vi "poly_asynch_wait_wait.vi"(4 "restart asynch wait? (F)":bool, 6 "check interval (50 ms)":u32=50, 8 "error in":errorcluster, 9 "timeout [ms]":i32, 10 "asynch wait ref in":T1) -> (0 "error out":errorcluster, 1 "timed out?":bool, 2 "asynch wait ref out":T1, 5 "remaining time":i32)   [LabVIEW 2015, in "_timing_tools_polys.lvlib"]
uses:
  _timing_tools_polys.lvlib
  asynch_wait_ref.ctl
  boolean_notifier.ctl
  poly_timing_tools_eco_plus.vi
  <vilib>/GPower/Timing/Library/Remaining/Remaining_ms.vi
  <vilib>/GPower/Timing/Library/Wait/Wait_ms.vi
  <vilib>/GPower/Error/Library/IsError.vi
  <vilib>/GPower/Timing/GPTiming.lvlib
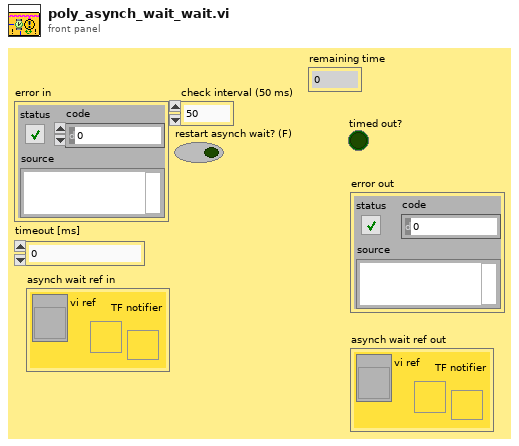
[diagram p1: front panel]
types:
  T1 = typedef "_timing_tools_polys.lvlib/asynch_wait_ref.ctl" = cluster{"vi ref":refnum<vi>, "TF notifier":T2}
  T2 = typedef "_timing_tools_polys.lvlib/boolean_notifier.ctl" = refnum<notifier>
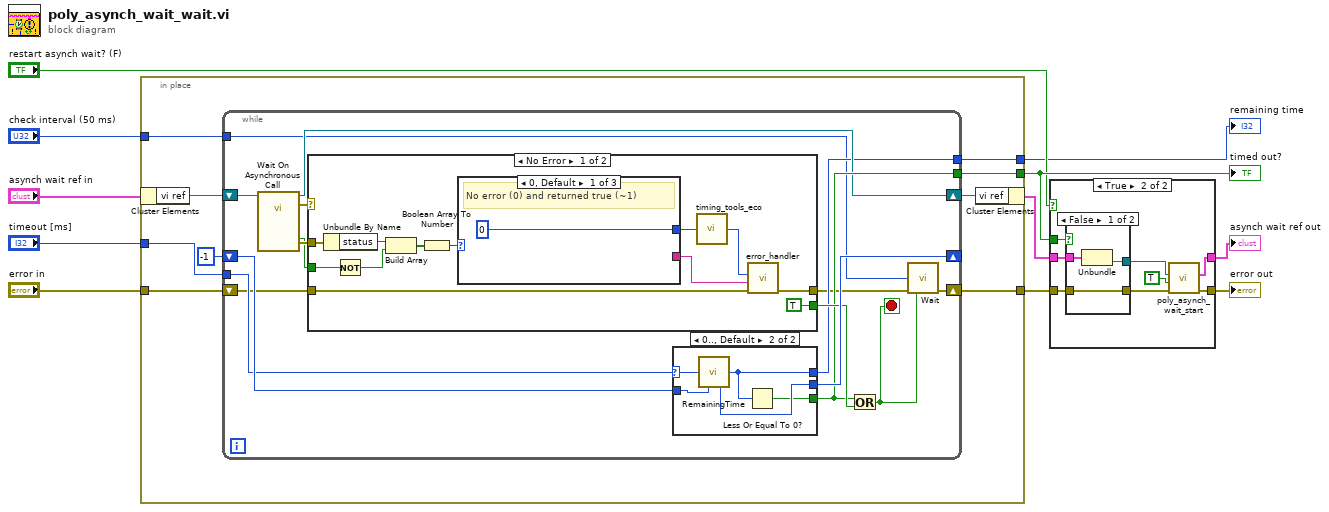
[diagram p0: block diagram]
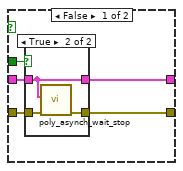
[diagram p2: hidden frame]
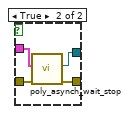
[diagram p4: hidden frame]
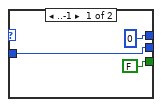
[diagram p5: hidden frame]
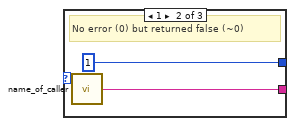
[diagram p6: hidden frame]
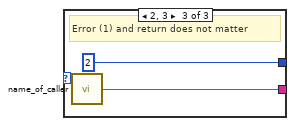
[diagram p7: hidden frame]
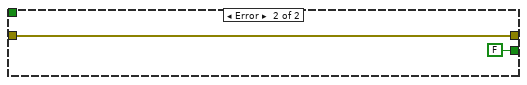
[diagram p8: hidden frame]
diagram:
  n1 = in-place {
    in-place-border: "timeout [ms]" -> [w18]
    in-place-border: [w17] -> w5
    in-place-border: "check interval (50 ms)" -> [w15]
    in-place-border: [w14] -> w3
    in-place-border: "error in" -> [w13]
    in-place-border: [w12] -> w1
    n2 = in-place-cluster #1("asynch wait ref in") -> ("vi ref"=w20:refnum<vi>)
    n3 = while {
      shift-right: [w32] -> _
      shift-left: i64 -1 ("Start time out") -> [w33]
      tunnel: w18 -> [w28]
      tunnel: [w30] -> w17
      shift-right: [w29] -> w16
      shift-left: w20 -> [w36]
      tunnel: w15 -> [w24]
      shift-right: [w22] -> w14
      shift-left: w13 -> [w26]
      tunnel: [w25] -> w12
      stop <- w21 stop-if-true
      n4 = call-by-ref "Wait On Asynchronous Call"(reference=w36) -> (reference out=w29:refnum<vi>, error out=w35:errorcluster, "Error out"=w34:errorcluster, "notification"=w27:bool)  [unwired: 9 in, 2 out]
      n5 = case shown="No Error" w35 {
        tunnel: w34 -> [w54 _]
        tunnel: [TRUE FALSE] -> w31
        tunnel: w27 -> [w50 _]
        tunnel: [w48 w62] -> w23
        tunnel: w26 -> [w55 w62]
        frame No Error {
          n6 = Unbundle By Name(w54) -> ("status"=w53:bool)
          n7 = Not(x=w50) -> (.not. x?=w49:bool)
          n8 = Build Array(w53, w49) -> (w52:bool[])
          n9 = Boolean Array To Number(Boolean array=w52) -> (number=w51:u32)
          n10 = case shown="0, Default" w51 {
            tunnel: [0 1 2] -> w46
            tunnel: [_ w58 w60] -> w47
            frame 0, Default {
              # "No error (0) and returned true (~1)"
            }
            frame 1 {
              # "No error (0) but returned false (~0)"
              n11 = call "name_of_caller.vi"() -> ("name of caller out"=w58:string)  [unwired: 4 in]
            }
            frame 2, 3 {
              # "Error (1) and return does not matter"
              n12 = call "name_of_caller.vi"() -> ("name of caller out"=w60:string)  [unwired: 4 in]
            }
          }
          n13 = call-poly "timing_tools_eco.vi"("code (w/out eco)"=w46) -> ("code (+ eco)"=w45:i32)  [unwired: 4 in]
          n14 = call "error_handler.vi"("error in (no error)"=w55, "name of caller in (you)"=w47, "code (0 = no error)"=w45) -> ("error out"=w48:errorcluster)  [unwired: 7 in, 1 out]
        }
        frame Error {
        }
      }
      n15 = case shown="0.., Default" w28 {
        selector: w28 -> [_ w41]
        tunnel: w33 -> [w39 w44]
        tunnel: [w39 w43] -> w32
        tunnel: [FALSE w42] -> w30
        tunnel: [0 ("Remaining time") w40] -> w25
        frame ..-1 {
        }
        frame 0.., Default {
          n16 = call-poly <vilib>:"RemainingTime.vi"("Time period target"=w41, "Start time in"=w44) -> ("Remaining time"=w40:i32, "Start time out"=w43:i64)  [unwired: 9 in, 3 out]
          n17 = Less Or Equal To 0?(x=w40) -> (x <= 0?=w42:bool)
        }
      }
      n18 = Or(x=w30, y=w31) -> (x .or. y?=w21:bool)
      n19 = call-poly <vilib>:"Wait.vi"("Time to wait"=w24, "Error in"=w23, "Skip wait?"=w21) -> ("Error out"=w22:errorcluster)  [unwired: 12 in]
    }
    n20 = in-place-cluster #1("vi ref"=w16) -> (w8:T1)
  }
  "timed out?" <- w5
  "remaining time" <- w1
  n21 = case shown="True" "restart asynch wait? (F)" {
    tunnel: w8 -> [w66 w78]
    tunnel: [w65 w77] -> w7
    tunnel: w3 -> [w68 w76]
    tunnel: [w67 w75] -> w6
    tunnel: w5 -> [w64 w74]
    frame False {
      n22 = case shown="True" w64 {
        tunnel: w66 -> [w69 w71]
        tunnel: w68 -> [w70 w73]
        tunnel: [w70 w72] -> w67
        tunnel: [w69 w71] -> w65
        frame False {
        }
        frame True {
          n23 = call "poly_asynch_wait_stop.vi"("error in"=w73, "asynch wait ref in"=w71) -> ("error out"=w72:errorcluster)  [unwired: 8 in, 1 out]
        }
      }
    }
    frame True {
      n24 = case shown="False" w74 {
        tunnel: [w82 w88] -> w80
        tunnel: [w83 w87] -> w79
        tunnel: w78 -> [w84 w86]
        tunnel: w76 -> [w82 w85]
        frame False {
          n25 = Unbundle(w84) -> ("TF notifier"=w83:T2)  [unwired: 1 out]
        }
        frame True {
          n26 = call "poly_asynch_wait_stop.vi"("error in"=w85, "asynch wait ref in"=w86) -> ("error out"=w88:errorcluster, "notifier"=w87:T2)  [unwired: 8 in]
        }
      }
      n27 = call "poly_asynch_wait_start.vi"("error in"=w80, "ignore previous (T)"=TRUE, "notifier (create)"=w79) -> ("error out"=w75:errorcluster, "asynch wait ref out"=w77:T1)  [unwired: 6 in, 1 out]
    }
  }
  "asynch wait ref out" <- w7
  "error out" <- w6
